vi "5.1-Parse Act Command.vi"(1 "data out":string) -> (0 "GUI":T1)   [LabVIEW 2010]
uses:
  4-High Neurons/4.0-Timing Badass.ctl
  6-OCU Neurons/6.1-Act.ctl
  6-OCU Neurons/6.1-UDP Saitek.ctl
  5.0-Global.vi
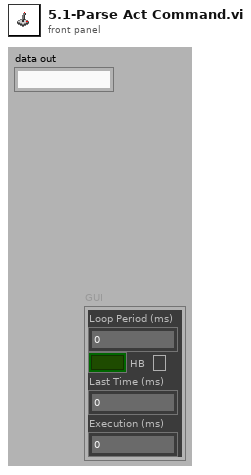
[diagram p1: front panel]
types:
  T1 = typedef "4.0-Timing Badass.ctl" = cluster{"Loop Period (ms)":u32, "HB":bool, "Last Time (ms)":u32, "Execution (ms)":u32}
  T2 = typedef "6.1-Act.ctl" = cluster{"6.1-Saitek Controller":T3, "Joystick Mode":bool, "Shutdown":bool, "Reset":bool, "Begin":bool}
  T3 = typedef "6.1-UDP Saitek.ctl" = cluster{"Stop":bool, "Setpoint":bool, "Run":bool, "Restart":bool, "Shutdown":bool, "Joystick\nMode 1":bool, "Joystick\nMode 2":bool, "Joystick \nMode 3":bool, "Joystick Mode 4":bool, "10":bool, "11":bool, "Pitch":sgl, "Roll":sgl, "Yaw":sgl, "Left":sgl, "Right":sgl}
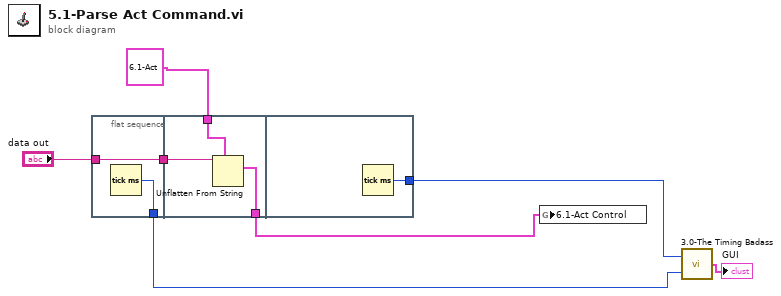
[diagram p0: block diagram]
diagram:
  n1 = flat-sequence {
    tunnel: "data out" -> [w8]
    tunnel: [w9] -> w4
    tunnel: [w8] -> w3
    tunnel: T2 {"6.1-Saitek Controller"={"Stop"=FALSE, "Setpoint"=FALSE, "Run"=FALSE, "Restart"=FALSE, "Shutdown"=FALSE, "Joystick\nMode 1"=FALSE, "Joystick\nMode 2"=FALSE, "Joystick \nMode 3"=FALSE, "Joystick Mode 4"=FALSE, "10"=FALSE, "11"=FALSE, "Pitch"=0.0, "Roll"=0.0, "Yaw"=0.0, "Left"=0.0, "Right"=0.0}, "Joystick Mode"=FALSE, "Shutdown"=FALSE, "Reset"=FALSE, "Begin"=FALSE} ("6.1-Act") -> [w11]
    tunnel: w3 -> [w12]
    tunnel: [w10] -> w1
    tunnel: [w13] -> w5
    frame #0 {
      n2 = Tick Count (ms)() -> (millisecond timer value=w9:u32)
    }
    frame #1 {
      n3 = Unflatten From String(type=w11, binary string=w12) -> (value=w10:T2)  [unwired: 3 in, 2 out]
    }
    frame #2 {
      n4 = Tick Count (ms)() -> (millisecond timer value=w13:u32)
    }
  }
  n5 = global write "5.0-Global.vi" "6.1-Act Control"(w1) -> ()
  n6 = call "3.0-The Timing Badass.vi"("Start"=w4, "End"=w5) -> ("Super Heart Beat"=→"GUI":T1)
